vi "Parse Value.vi"(8 "error in (no error)":errorcluster, 10 "Index In":i32, 11 "JSON String":string) -> (0 "error out":errorcluster, 2 "Index Out":i32, 3 "JSON out":refnum<class "JSON Value.lvclass">)   [LabVIEW 2016, in "JSON Value.lvclass"]
uses:
  JSON Value.lvclass
  JSON Boolean/New JSON Boolean.vi
  JSON Datatype/New JSON Null.vi
  Errors/Errors.ctl
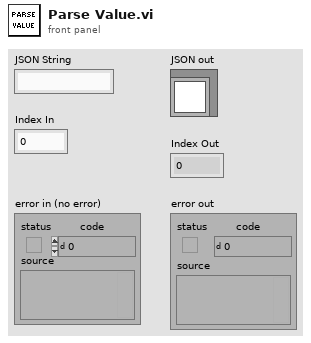
[diagram p1: front panel]
types:
  T1 = typedef "JSON Value.lvclass/Errors.ctl" = enum16{"No key", "Key path type", "Array OOB", "Type Mismatch", "Invalid Token"}
  T2 = typedef "JSON Value.lvclass/Token Type.ctl" = enum16{"NONE", "CURLY_OPEN", "CURLY_CLOSE", "SQUARED_OPEN", "SQUARED_CLOSE", "COLON", "COMMA", "STRING", "NUMBER", "TRUE", "FALSE", "NULL"}
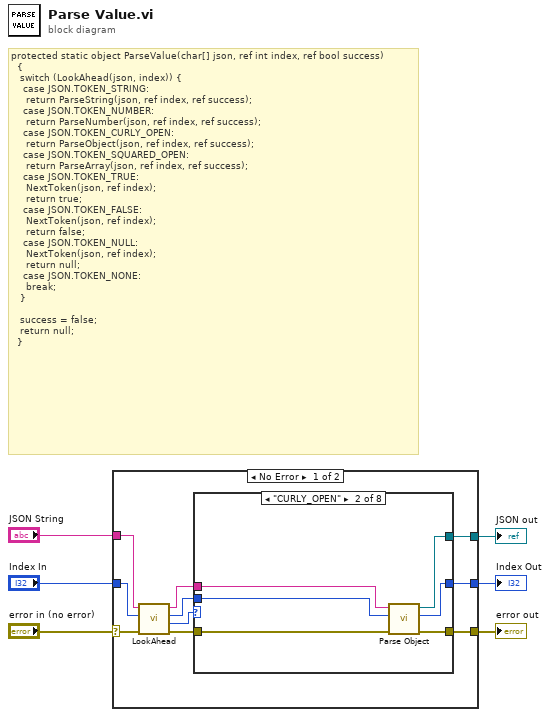
[diagram p0: block diagram]
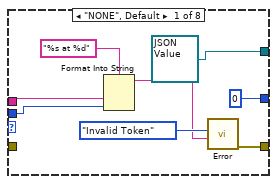
[diagram p2: hidden frame]
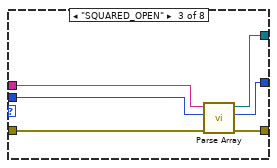
[diagram p3: hidden frame]
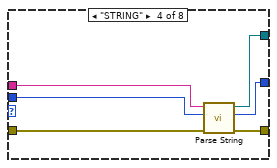
[diagram p4: hidden frame]
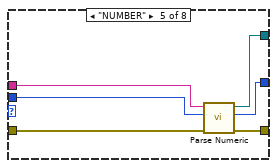
[diagram p5: hidden frame]
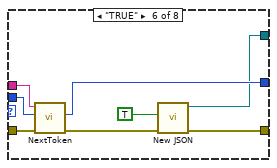
[diagram p6: hidden frame]
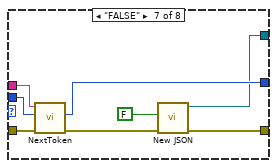
[diagram p7: hidden frame]
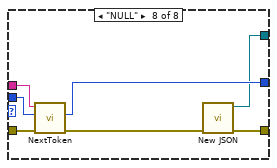
[diagram p8: hidden frame]
diagram:
  # "protected static object ParseValue(char[] json, ref int index, ref bool success)\n\t\t{\n\t\t\tswitch (LookAhead(json, index)) {\n\t\t\t\tcase JSON.TOKEN_STRING:\n\t\t\t\t\treturn ParseString(json, ref index, ref success);\n\t\t\t\tcase JSON.TOKEN_NUMBER:\n\t\t\t\t\treturn ParseNumber(json, ref index, ref success);\n\t\t\t\tcase JSON.TOKEN_CURLY_OPEN:\n\t\t\t\t\treturn ParseObject(json, ref index, ref success);\n\t\t\t\tcase JSON.TOKEN_SQUARED_OPEN:\n\t\t\t\t\treturn ParseArray(json, ref index, ref success);\n\t\t\t\tcase JSON.TOKEN_TRUE:\n\t\t\t\t\tNextToken(json, ref index);\n\t\t\t\t\treturn true;\n\t\t\t\tcase JSON.TOKEN_FALSE:\n\t\t\t\t\tNextToken(json, ref index);\n\t\t\t\t\treturn false;\n\t\t\t\tcase JSON.TOKEN_NULL:\n\t\t\t\t\tNextToken(json, ref index);\n\t\t\t\t\treturn null;\n\t\t\t\tcase JSON.TOKEN_NONE:\n\t\t\t\t\tbreak;\n\t\t\t}\n\n\t\t\tsuccess = false;\n\t\t\treturn null;\n\t\t}"
  n1 = case shown="No Error" "error in (no error)" {
    selector: "error in (no error)" -> [w16 w72]
    tunnel: [w14 w72] -> w5
    tunnel: "JSON String" -> [w10 _]
    tunnel: "Index In" -> [w9 _]
    tunnel: [w8 _] -> w1
    tunnel: [w7 _] -> w2
    frame No Error {
      n2 = call "LookAhead.vi"("error in (no error)"=w16, "Index"=w9, "JSON String"=w10) -> ("error out"=w15:errorcluster, "TOKEN"=w13:T2, "Index Passthrough"=w11:i32, "JSON String Passthrough"=w12:string)  [unwired: 5 in]
      n3 = case shown="\"CURLY_OPEN\"" w13 {
        tunnel: w15 -> [_ w28 w34 w40 w46 w53 w62 w68]
        tunnel: [w23 w27 w33 w39 w45 w50 w59 w66] -> w14
        tunnel: [refnum<class "JSON Value.lvclass"> refnum ("JSON Object in") w25 w31 w37 w43 w49 w57 w65] -> w8
        tunnel: w12 -> [w20 w29 w36 w42 w48 w56 w60 w70]
        tunnel: w11 -> [w19 w30 w35 w41 w47 w55 w61 w69]
        tunnel: [0 ("Index Out") w26 w32 w38 w44 w54 w63 w67] -> w7
        frame "NONE", Default {
          n4 = Format Into String(format string="%s at %d", w20, w19) -> (resulting string=w18:string)  [unwired: 2 in, 1 out]
          n5 = call "Error.vi"("Data"=w18, 9:Errors."Invalid Token") -> ("error out"=w23:errorcluster)  [unwired: 8 in]
        }
        frame "CURLY_OPEN" {
          n6 = call "Parse Object.vi"("error in (no error)"=w28, "Index In"=w30, "JSON String"=w29) -> ("error out"=w27:errorcluster, "Index Out"=w26:i32, "JSON Object out"=w25:refnum<class "JSON Value.lvclass">)  [unwired: 6 in]
        }
        frame "SQUARED_OPEN" {
          n7 = call "Parse Array.vi"("error in (no error)"=w34, "Index In"=w35, "JSON String"=w36) -> ("error out"=w33:errorcluster, "Index Out"=w32:i32, "JSON out"=w31:refnum<class "JSON Value.lvclass">)  [unwired: 6 in]
        }
        frame "STRING" {
          n8 = call "Parse String.vi"("error in (no error)"=w40, "Index In"=w41, "JSON String"=w42) -> ("error out"=w39:errorcluster, "Index Out"=w38:i32, "JSON out"=w37:refnum<class "JSON Value.lvclass">)  [unwired: 5 in, 1 out]
        }
        frame "NUMBER" {
          n9 = call "Parse Numeric.vi"("error in (no error)"=w46, "Index In"=w47, "JSON String"=w48) -> ("error out"=w45:errorcluster, "Index Out"=w44:i32, "JSON out"=w43:refnum<class "JSON Value.lvclass">)  [unwired: 6 in]
        }
        frame "TRUE" {
          n10 = call "NextToken.vi"("error in (no error)"=w53, "Index In"=w55, "JSON String"=w56) -> ("error out"=w51:errorcluster, "Index Out"=w54:i32)  [unwired: 5 in, 2 out]
          n11 = call-poly "New JSON.vi"("error in (no error)"=w51, "value"=TRUE) -> ("error out"=w50:errorcluster, "JSON Boolean out"=w49:refnum<class "JSON Value.lvclass">)  [unwired: 8 in]
        }
        frame "FALSE" {
          n12 = call "NextToken.vi"("error in (no error)"=w62, "Index In"=w61, "JSON String"=w60) -> ("error out"=w64:errorcluster, "Index Out"=w63:i32)  [unwired: 5 in, 2 out]
          n13 = call-poly "New JSON.vi"("error in (no error)"=w64, "value"=FALSE) -> ("error out"=w59:errorcluster, "JSON Boolean out"=w57:refnum<class "JSON Value.lvclass">)  [unwired: 8 in]
        }
        frame "NULL" {
          n14 = call "NextToken.vi"("error in (no error)"=w68, "Index In"=w69, "JSON String"=w70) -> ("error out"=w71:errorcluster, "Index Out"=w67:i32)  [unwired: 5 in, 2 out]
          n15 = call-poly "New JSON.vi"("error in (no error)"=w71) -> ("error out"=w66:errorcluster, "JSON Null out"=w65:refnum<class "JSON Value.lvclass">)  [unwired: 9 in]
        }
      }
    }
    frame Error {
    }
  }
  "error out" <- w5
  "Index Out" <- w2
  "JSON out" <- w1
